vi "Launch Connection Handler.vi"(8 "error in (no error)":errorcluster, 11 "Server in":refnum<class "Server.lvclass">) -> (0 "error out":errorcluster, 3 "Server out":refnum<class "Server.lvclass">)   [LabVIEW 2013, in "MQTT Server.lvlib" / "Server.lvclass"]
uses:
  Server.lvclass
  MQTT_Base/Base Class/MQTT_Base.lvclass/MQTT_Base.ctl
  Server.lvclass/Server.ctl
  MQTT_Connection/Connection/Connection.lvclass
  <vilib>/LabVIEW Open Source Project/MQTT Control Packets/Control Packets/ControlPacket/ControlPacket.lvclass
  MQTT_Connection/ConnectionHandler/ConnectionHandler.lvclass
  MQTT_Base/Base Class/MQTT_Base.lvclass
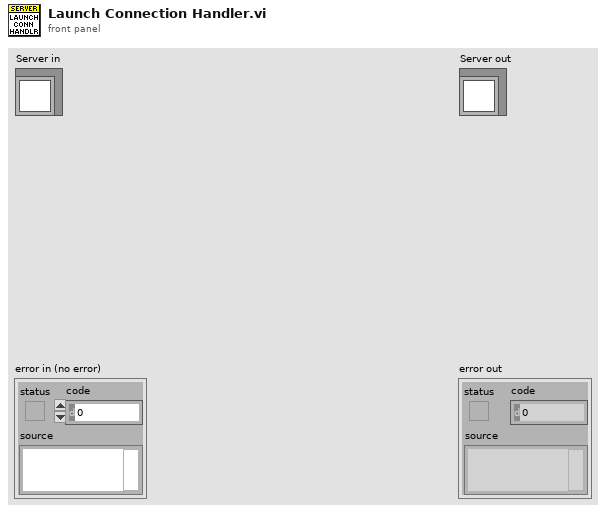
[diagram p1: front panel]
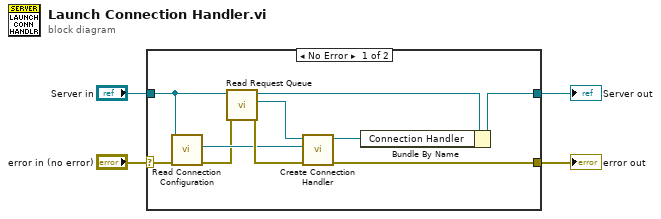
[diagram p0: block diagram]
diagram:
  n1 = case shown="No Error" "error in (no error)" {
    selector: "error in (no error)" -> [w6 w16]
    tunnel: [w9 w16] -> w3
    tunnel: [w14 w15] -> w1
    tunnel: "Server in" -> [w8 w15]
    frame No Error {
      n2 = call "Read Connection Configuration.vi"("error in (no error)"=w6, "MQTT_Base in"=w8) -> ("error out"=w5:errorcluster, "Connection Configuration"=w7:refnum<class "Connection.lvclass">)  [unwired: 7 in, 1 out]
      n3 = call "Read Request Queue.vi"("error in (no error)"=w5, "MQTT_Base in"=w8) -> ("error out"=w11:errorcluster, "Request"=w12:refnum<queue>, "MQTT_Base out"=w13:refnum<class "Server.lvclass">)  [unwired: 7 in]
      n4 = call "Create Connection Handler.vi"("error in (no error)"=w11, "Connection Configuration"=w7, "Request"=w12) -> ("error out"=w9:errorcluster, "ConnectionHandler"=w10:refnum<class "ConnectionHandler.lvclass">)  [unwired: 7 in]
      n5 = Bundle By Name(cluster=w13, "Connection Handler"=w10) -> (w14:refnum<class "Server.lvclass">)
    }
    frame Error {
    }
  }
  "error out" <- w3
  "Server out" <- w1
